vi "superhetero.vi"() -> ()   [LabVIEW 2009]
uses:
  <vilib>/Analysis/NI_AALBase.lvlib
panel:
  in  "数値 2":dbl
  in  "数値":dbl
  out "歪み率":dbl
  out "出力":cluster{dbl[], dbl[]}(graph) caption="XYグラフ"
  out "送信波":cluster{dbl[], dbl[]}(graph)
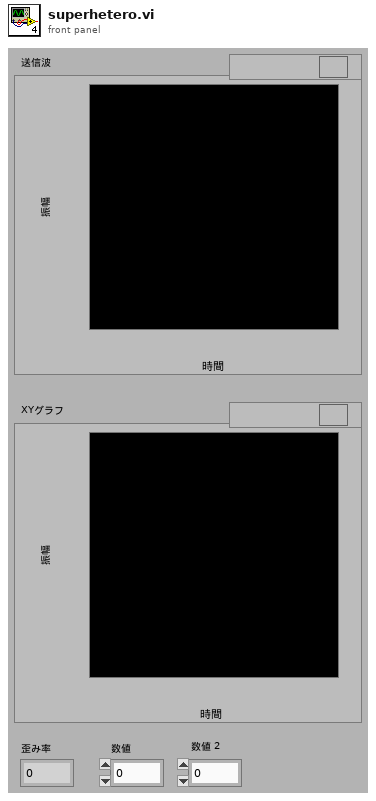
[diagram p1: front panel]
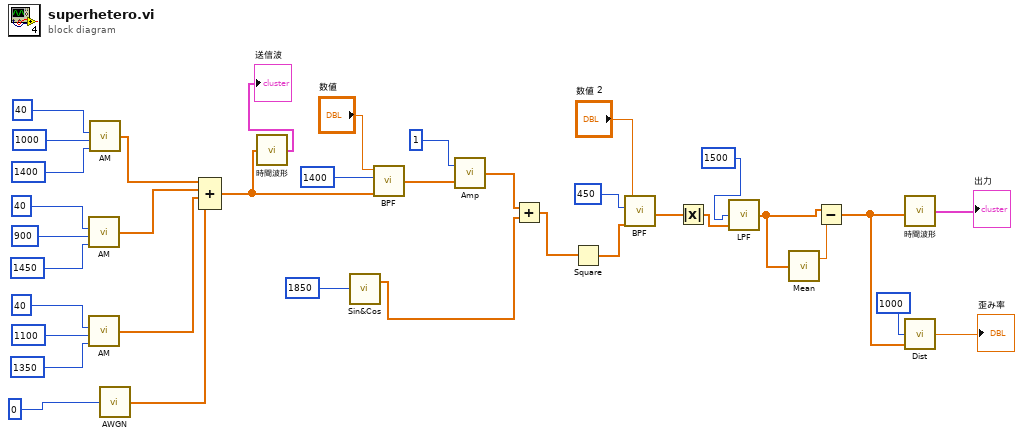
[diagram p0: block diagram]
diagram:
  n1 = call "AM.vi"("変調度 [%]"=40, "変調周波数 [Hz]"=900, "搬送波周波数 [kHz]"=1450) -> ("変調波"=w26:dbl[])  [unwired: 2 in]
  n2 = call "AM.vi"("変調度 [%]"=40, "変調周波数 [Hz]"=1100, "搬送波周波数 [kHz]"=1350) -> ("変調波"=w25:dbl[])  [unwired: 2 in]
  n3 = call "AM.vi"("変調度 [%]"=40, "変調周波数 [Hz]"=1000, "搬送波周波数 [kHz]"=1400) -> ("変調波"=w27:dbl[])  [unwired: 2 in]
  n4 = call "AWGN.vi"("振幅値"=0) -> ("出力"=w24:dbl[])
  n5 = Compound Arithmetic op=ADD(w27, w26, w25, w24) -> (w21:dbl[])
  n6 = call "時間波形.vi"("入力"=w21) -> ("時間波形"=→"送信波":cluster{dbl[], dbl[]})
  n7 = call "Sin&Cos.vi"("周波数[kHz]"=1850) -> ("sin"=w5:dbl[])  [unwired: 1 out]
  n8 = call "BPF.vi"("X"=w21, "中心周波数 [kHz]"=1400, "Q"="数値") -> ("BPF出力"=w7:dbl[])  [unwired: 1 in]
  n9 = call "Amp.vi"("入力"=w7, "増幅率"=1) -> ("出力"=w6:dbl[])
  n10 = Add(x=w6, y=w5) -> (x+y=w4:dbl[])
  n11 = Square(x=w4) -> (x^2=w3:dbl[])
  n12 = call "BPF.vi"("X"=w3, "中心周波数 [kHz]"=450, "Q"="数値 2") -> ("BPF出力"=w14:dbl[])  [unwired: 1 in]
  n13 = Absolute Value(x=w14) -> (abs(x)=w13:dbl[])
  n14 = call "LPF.vi"("入力"=w13, "カットオフ周波数 [Hz]"=1500) -> ("LPF出力"=w11:dbl[])  [unwired: 1 in]
  n15 = call <vilib>:"Mean.vi"("X"=w11) -> ("mean"=w12:dbl)  [unwired: 1 out]
  n16 = Subtract(x=w11, y=w12) -> (x-y=w10:dbl[])
  n17 = call "時間波形.vi"("入力"=w10) -> ("時間波形"=→"出力":cluster{dbl[], dbl[]})
  n18 = call "Dist.vi"("入力"=w10, "基本周波数 [Hz]"=1000) -> ("ひずみ率"=→"歪み率":dbl)  [unwired: 1 in]
